vi "Auto1-CrossBaseline.vi"(5 "End By Time":timestamp, 7 "Start Time":timestamp, 11 "Game Data":string) -> (3 "Actual End Time":timestamp)   [LabVIEW 2017]
uses:
  AutoGeneralInput.ctl
  DriveAutoInput.ctl
  DriveAutoType.ctl
  DriveAutoDirections.ctl
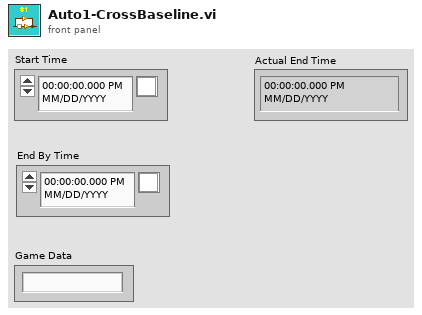
[diagram p1: front panel]
types:
  T1 = typedef "AutoGeneralInput.ctl" = cluster{"Start by (s)":dbl, "End by (s)":dbl, "Auto Start Time":timestamp}
  T2 = typedef "DriveAutoInput.ctl" = cluster{"DriveAutoMode":T3, "ModeParameters":cluster{"Arc Difference":dbl, "Angle":dbl, "Linear Value":dbl}, "LinearControlMethod":enum16{"Feedback", "Time"}, "Directions":T4}
  T3 = typedef "DriveAutoType.ctl" = enum16{"Straight", "Spin", "Arc"}
  T4 = typedef "DriveAutoDirections.ctl" = cluster{"Forward/Reverse":enum16{"Forward", "Reverse"}, "Right/Left":enum16{"Right/CW", "Left/CCW"}}
  T5 = typedef "AutoGeneralOutput.ctl" = cluster{"Ended Safe?":bool, "True Start (s)":dbl, "True End (s)":dbl}
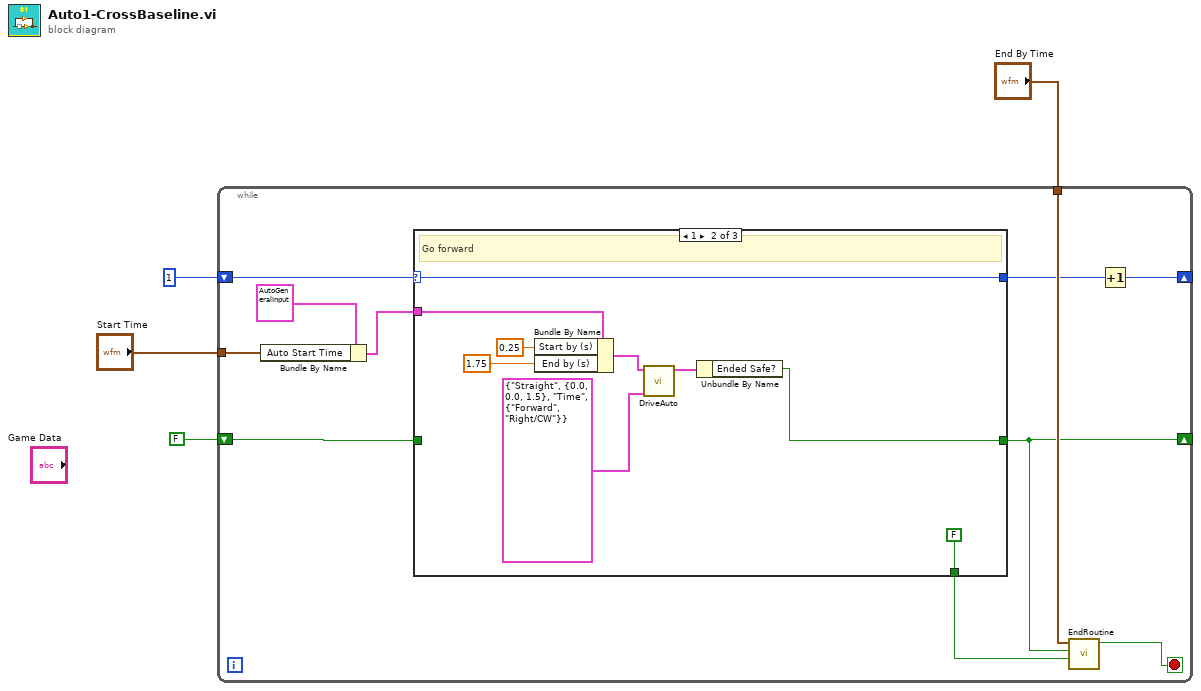
[diagram p0: block diagram]
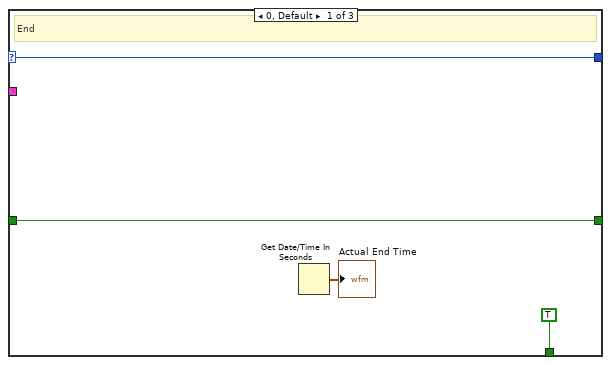
[diagram p2: hidden frame]
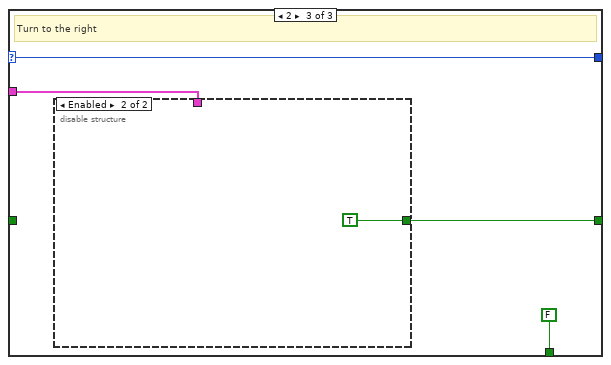
[diagram p3: hidden frame]
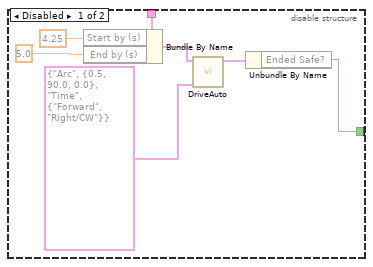
[diagram p4: hidden frame]
diagram:
  n1 = while {
    tunnel: "Start Time" -> [w8]
    tunnel: "End By Time" -> [w15]
    shift-right: [w5] -> _
    shift-left: 1 -> [w14]
    shift-right: [w10] -> _
    shift-left: FALSE ("Ended Safe?") -> [w11]
    stop <- w12 stop-if-true
    n2 = Bundle By Name(cluster=T1 {"Start by (s)"=1.0, "End by (s)"=4.0, "Auto Start Time"=timestamp(0 s since 1904-01-01)} ("GeneralAutoInput"), "Auto Start Time"=w8) -> (w6:T1)
    n3 = case shown="1" w14 {
      selector: w14 -> [w16 w20 w29]
      tunnel: [w16 w20 w29] -> w13
      tunnel: w6 -> [_ w27 w32]
      tunnel: [w19 w22 w31] -> w10
      tunnel: w11 -> [w19 _ _]
      tunnel: [TRUE ("Ended Safe?") FALSE ("Ended Safe?") FALSE ("Ended Safe?")] -> w9
      frame 0, Default {
        # "End"
        n4 = Get Date/Time In Seconds() -> (seconds since 1Jan1904=→"Actual End Time":timestamp)
      }
      frame 1 {
        # "Go forward"
        n5 = Bundle By Name(cluster=w27, "Start by (s)"=0.25, "End by (s)"=1.75) -> (w23:T1)
        n6 = call "DriveAuto.vi"("DriveAutoInput"=T2 {"DriveAutoMode"=enum."Straight", "ModeParameters"={"Arc Difference"=0.0, "Angle"=0.0, "Linear Value"=1.5}, "LinearControlMethod"=enum."Time", "Directions"={"Forward/Reverse"=enum."Forward", "Right/Left"=enum."Right/CW"}}, "GeneralAutoInput"=w23) -> ("AutoGeneralOut"=w24:T5)  [unwired: 9 in]
        n7 = Unbundle By Name(w24) -> ("Ended Safe?"=w22:bool)
      }
      frame 2 {
        # "Turn to the right"
        n8 = disable-structure shown="Enabled" {
          disable-tunnel: w32 -> [w38 _]
          disable-tunnel: [w33 TRUE] -> w31
          frame Disabled {
            n9 = Bundle By Name(cluster=w38, "Start by (s)"=4.25, "End by (s)"=5.0) -> (w34:T1)
            n10 = call "DriveAuto.vi"("DriveAutoInput"=T2 {"DriveAutoMode"=enum."Arc", "ModeParameters"={"Arc Difference"=0.5, "Angle"=90.0, "Linear Value"=0.0}, "LinearControlMethod"=enum."Time", "Directions"={"Forward/Reverse"=enum."Forward", "Right/Left"=enum."Right/CW"}}, "GeneralAutoInput"=w34) -> ("AutoGeneralOut"=w35:T5)  [unwired: 9 in]
            n11 = Unbundle By Name(w35) -> ("Ended Safe?"=w33:bool)
          }
          frame Enabled {
          }
        }
      }
    }
    n12 = call "EndRoutine.vi"("End?"=w9, "Ended Safe?"=w10, "End Time"=w15) -> ("Stop?"=w12:bool)  [unwired: 8 in]
    n13 = Increment(x=w13) -> (x+1=w5:i32)
  }
